vi "GeoData.vi"() -> ()   [LabVIEW 2017] (continued)
County\tH1\n40241\t21111\tLouisville\tKY\tJefferson County\tH1\n40207\t21111\tLouisville\tKY\tJefferson County\tH1\n40242\t21111\tLouisville\tKY\tJefferson County\tH1\n40272\t21111\tLouisville\tKY\tJefferson County\tH1\n40210\t21111\tLouisville\tKY\tJefferson County\tH1\n40270\t21111\tLouisville\tKY\tJefferson County\tH1\n40025\t21111\tGlenview\tKY\tJefferson County\tH1\n40027\t21111\tHarrods creek\tKY\tJefferson County\tH1\n40225\t21111\tLouisville\tKY\tJefferson County\tH1\n40281\t21111\tLouisville\tKY\tJefferson County\tH1\n40214\t21111\tLouisville\tKY\tJefferson County\tH1\n40257\t21111\tLouisville\tKY\tJefferson County\tH1\n40251\t21111\tLouisville\tKY\tJefferson County\tH1\n40292\t21111\tLouisville\tKY\tJefferson County\tH1\n40289\t21111\tLouisville\tKY\tJefferson County\tH1\n40177\t21111\tWest point\tKY\tJefferson County\tH1\n40216\t21111\tLouisville\tKY\tJefferson County\tH1\n40256\t21111\tLouisville\tKY\tJefferson County\tH1\n40291\t21111\tLouisville\tKY\tJefferson County\tH1\n40218\t21111\tLouisville\tKY\tJefferson County\tH1\n40217\t21111\tLouisville\tKY\tJefferson County\tH1\n40204\t21111\tLouisville\tKY\tJefferson County\tH1\n40056\t21111\tPewee valley\tKY\tJefferson County\tH1\n40250\t21111\tLouisville\tKY\tJefferson County\tH1\n40261\t21111\tLouisville\tKY\tJefferson County\tH1\n40018\t21111\tEastwood\tKY\tJefferson County\tH1\n40266\t21111\tLouisville\tKY\tJefferson County\tH1\n40285\t21111\tLouisville\tKY\tJefferson County\tH1\n40047\t21111\tMount washington\tKY\tJefferson County\tH1\n40059\t21111\tProspect\tKY\tJefferson County\tH1\n40219\t21111\tLouisville\tKY\tJefferson County\tH1\n40258\t21111\tLouisville\tKY\tJefferson County\tH1\n40205\t21111\tLouisville\tKY\tJefferson County\tH1\n40233\t21111\tLouisville\tKY\tJefferson County\tH1\n40255\t21111\tLouisville\tKY\tJefferson County\tH1\n40201\t21111\tLouisville\tKY\tJefferson County\tH1\n40202\t21111\tLouisville\tKY\tJefferson County\tH1\n40023\t21111\tFisherville\tKY\tJefferson County\tH1\n40245\t21111\tLouisville\tKY\tJefferson County\tH1\n40206\t21111\tLouisville\tKY\tJefferson County\tH1\n40228\t21111\tLouisville\tKY\tJefferson County\tH1\n40252\t21111\tLouisville\tKY\tJefferson County\tH1\n40268\t21111\tLouisville\tKY\tJefferson County\tH1\n40014\t21111\tCrestwood\tKY\tJefferson County\tH1\n40109\t21111\tBrooks\tKY\tJefferson County\tH1\n40118\t21111\tFairdale\tKY\tJefferson County\tH1\n40203\t21111\tLouisville\tKY\tJefferson County\tH1\n40211\t21111\tLouisville\tKY\tJefferson County\tH1\n40220\t21111\tLouisville\tKY\tJefferson County\tH1\n40243\t21111\tLouisville\tKY\tJefferson County\tH1\n40212\t21111\tLouisville\tKY\tJefferson County\tH1\n40215\t21111\tLouisville\tKY\tJefferson County\tH1\n40299\t21111\tLouisville\tKY\tJefferson County\tH1\n40253\t21111\tLouisville\tKY\tJefferson County\tH1\n40232\t21111\tLouisville\tKY\tJefferson County\tH1\n40283\t21111\tLouisville\tKY\tJefferson County\tH1\n40231\t21111\tLouisville\tKY\tJefferson County\tH1\n40223\t21111\tLouisville\tKY\tJefferson County\tH1\n40222\t21111\tLouisville\tKY\tJefferson County\tH1\n40208\t21111\tLouisville\tKY\tJefferson County\tH1\n40213\t21111\tLouisville\tKY\tJefferson County\tH1\n40221\t21111\tLouisville\tKY\tJefferson County\tH1\n40209\t21111\tLouisville\tKY\tJefferson County\tH1\n40383\t21113\tVersailles\tKY\tJessamine County\tH1\n40390\t21113\tWilmore\tKY\tJessamine County\tH1\n40340\t21113\tNicholasville\tKY\tJessamine County\tH1\n40515\t21113\tLexington\tKY\tJessamine County\tH1\n40339\t21113\tKeene\tKY\tJessamine County\tH1\n40356\t21113\tNicholasville\tKY\tJessamine County\tH1\n41255\t21115\tSitka\tKY\tJohnson County\tH1\n41240\t21115\tPaintsville\tKY\tJohnson County\tH1\n41238\t21115\tOil springs\tKY\tJohnson County\tH1\n41226\t21115\tKeaton\tKY\tJohnson County\tH1\n41256\t21115\tStaffordsville\tKY\tJohnson County\tH1\n41254\t21115\tRiver\tKY\tJohnson County\tH1\n41268\t21115\tWest van lear\tKY\tJohnson County\tH1\n41274\t21115\tWittensville\tKY\tJohnson County\tH1\n41465\t21115\tSalyersville\tKY\tJohnson County\tH1\n41219\t21115\tFlatgap\tKY\tJohnson County\tH1\n41159\t21115\tMartha\tKY\tJohnson County\tH1\n41260\t21115\tThelma\tKY\tJohnson County\tH1\n41204\t21115\tBoons camp\tKY\tJohnson County\tH1\n41265\t21115\tVan lear\tKY\tJohnson County\tH1\n41271\t21115\tWilliamsport\tKY\tJohnson County\tH1\n41257\t21115\tStambaugh\tKY\tJohnson County\tH1\n41263\t21115\tTutor key\tKY\tJohnson County\tH1\n41232\t21115\tLowmansville\tKY\tJohnson County\tH1\n41222\t21115\tHagerhill\tKY\tJohnson County\tH1\n41216\t21115\tEast point\tKY\tJohnson County\tH1\n41234\t21115\tMeally\tKY\tJohnson County\tH1\n41017\t21117\tFt mitchell\tKY\tKenton County\tH1\n41033\t21117\tDe mossville\tKY\tKenton County\tH1\n41015\t21117\tLatonia\tKY\tKenton County\tH1\n41018\t21117\tErlanger\tKY\tKenton County\tH1\n41030\t21117\tCrittenden\tKY\tKenton County\tH1\n41011\t21117\tCovington\tKY\tKenton County\tH1\n41063\t21117\tMorning view\tKY\tKenton County\tH1\n41053\t21117\tKenton\tKY\tKenton County\tH1\n41042\t21117\tFlorence\tKY\tKenton County\tH1\n41016\t21117\tCovington\tKY\tKenton County\tH1\n41094\t21117\tWalton\tKY\tKenton County\tH1\n41014\t21117\tCovington\tKY\tKenton County\tH1\n41012\t21117\tCovington\tKY\tKenton County\tH1\n41051\t21117\tIndependence\tKY\tKenton County\tH1\n45999\t21117\tCincinnati\tKY\tKenton County\tH1\n41339\t21119\tJackson\tKY\tKnott County\tH1\n41772\t21119\tVest\tKY\tKnott County\tH1\n41862\t21119\tTopmost\tKY\tKnott County\tH1\n41804\t21119\tBlackey\tKY\tKnott County\tH1\n41861\t21119\tRaven\tKY\tKnott County\tH1\n41859\t21119\tDema\tKY\tKnott County\tH1\n41722\t21119\tBulan\tKY\tKnott County\tH1\n41773\t21119\tVicco\tKY\tKnott County\tH1\n41828\t21119\tKite\tKY\tKnott County\tH1\n41725\t21119\tCarrie\tKY\tKnott County\tH1\n41743\t21119\tFisty\tKY\tKnott County\tH1\n41630\t21119\tGarrett\tKY\tKnott County\tH1\n41839\t21119\tMousie\tKY\tKnott County\tH1\n41834\t21119\tLittcarr\tKY\tKnott County\tH1\n41759\t21119\tSassafras\tKY\tKnott County\tH1\n41822\t21119\tHindman\tKY\tKnott County\tH1\n41701\t21119\tHazard\tKY\tKnott County\tH1\n41640\t21119\tHueysville\tKY\tKnott County\tH1\n41740\t21119\tEmmalena\tKY\tKnott County\tH1\n41847\t21119\tRedfox\tKY\tKnott County\tH1\n41836\t21119\tMallie\tKY\tKnott County\tH1\n41843\t21119\tPine top\tKY\tKnott County\tH1\n41817\t21119\tGarner\tKY\tKnott County\tH1\n41844\t21119\tPippa passes\tKY\tKnott County\tH1\n41831\t21119\tLeburn\tKY\tKnott County\tH1\n40903\t21121\tArtemus\tKY\tKnox County\tH1\n40982\t21121\tScalf\tKY\tKnox County\tH1\n40734\t21121\tGray\tKY\tKnox County\tH1\n40953\t21121\tHinkle\tKY\tKnox County\tH1\n40935\t21121\tFlat lick\tKY\tKnox County\tH1\n40997\t21121\tWalker\tKY\tKnox County\tH1\n40701\t21121\tCorbin\tKY\tKnox County\tH1\n40939\t21121\tFourmile\tKY\tKnox County\tH1\n40943\t21121\tGirdler\tKY\tKnox County\tH1\n40906\t21121\tBarbourville\tKY\tKnox County\tH1\n40923\t21121\tCannon\tKY\tKnox County\tH1\n40946\t21121\tGreen road\tKY\tKnox County\tH1\n40759\t21121\tRockholds\tKY\tKnox County\tH1\n40771\t21121\tWoodbine\tKY\tKnox County\tH1\n40915\t21121\tBimble\tKY\tKnox County\tH1\n40962\t21121\tManchester\tKY\tKnox County\tH1\n40763\t21121\tSiler\tKY\tKnox County\tH1\n40921\t21121\tBryants store\tKY\tKnox County\tH1\n40949\t21121\tHeidrick\tKY\tKnox County\tH1\n40995\t21121\tTrosper\tKY\tKnox County\tH1\n40051\t21123\tNew haven\tKY\tLarue County\tH1\n42716\t21123\tBuffalo\tKY\tLarue County\tH1\n42748\t21123\tHodgenville\tKY\tLarue County\tH1\n42757\t21123\tMagnolia\tKY\tLarue County\tH1\n40052\t21123\tNew hope\tKY\tLarue County\tH1\n42776\t21123\tSonora\tKY\tLarue County\tH1\n42764\t21123\tMount sherman\tKY\tLarue County\tH1\n42718\t21123\tCampbellsville\tKY\tLarue County\tH1\n42784\t21123\tUpton\tKY\tLarue County\tH1\n40740\t21125\tLily\tKY\tLaurel County\tH1\n40734\t21125\tGray\tKY\tLaurel County\tH1\n40701\t21125\tCorbin\tKY\tLaurel County\tH1\n40402\t21125\tAnnville\tKY\tLaurel County\tH1\n40729\t21125\tEast bernstadt\tKY\tLaurel County\tH1\n40906\t21125\tBarbourville\tKY\tLaurel County\tH1\n40755\t21125\tPittsburg\tKY\tLaurel County\tH1\n40744\t21125\tLondon\tKY\tLaurel County\tH1\n40741\t21125\tLondon\tKY\tLaurel County\tH1\n40962\t21125\tManchester\tKY\tLaurel County\tH1\n40750\t21125\tLondon\tKY\tLaurel County\tH1\n40456\t21125\tMount vernon\tKY\tLaurel County\tH1\n40737\t21125\tKeavy\tKY\tLaurel County\tH1\n40724\t21125\tBush\tKY\tLaurel County\tH1\n41124\t21127\tBlaine\tKY\tLawrence County\tH1\n41201\t21127\tAdams\tKY\tLawrence County\tH1\n41254\t21127\tRiver\tKY\tLawrence County\tH1\n41132\t21127\tDenton\tKY\tLawrence County\tH1\n41143\t21127\tGrayson\tKY\tLawrence County\tH1\n41159\t21127\tMartha\tKY\tLawrence County\tH1\n41180\t21127\tWebbville\tKY\tLawrence County\tH1\n41232\t21127\tLowmansville\tKY\tLawrence County\tH1\n41181\t21127\tWillard\tKY\tLawrence County\tH1\n41160\t21127\tMazie\tKY\tLawrence County\tH1\n41129\t21127\tCatlettsburg\tKY\tLawrence County\tH1\n41230\t21127\tLouisa\tKY\tLawrence County\tH1\n41264\t21127\tUlysses\tKY\tLawrence County\tH1\n41339\t21129\tJackson\tKY\tLee County\tH1\n41397\t21129\tZoe\tKY\tLee County\tH1\n41311\t21129\tBeattyville\tKY\tLee County\tH1\n41314\t21129\tBooneville\tKY\tLee County\tH1\n40336\t21129\tIrvine\tKY\tLee County\tH1\n41368\t21129\tSaint helens\tKY\tLee County\tH1\n41301\t21129\tCampton\tKY\tLee County\tH1\n41347\t21129\tLone\tKY\tLee County\tH1\n41365\t21129\tRogers\tKY\tLee County\tH1\n40858\t21131\tMozelle\tKY\tLeslie County\tH1\n41764\t21131\tSmilax\tKY\tLeslie County\tH1\n40914\t21131\tBig creek\tKY\tLeslie County\tH1\n41762\t21131\tSizerock\tKY\tLeslie County\tH1\n41723\t21131\tBusy\tKY\tLeslie County\tH1\n41777\t21131\tYeaddiss\tKY\tLeslie County\tH1\n40816\t21131\tChappell\tKY\tLeslie County\tH1\n41766\t21131\tThousandsticks\tKY\tLeslie County\tH1\n40818\t21131\tCoalgood\tKY\tLeslie County\tH1\n40803\t21131\tAsher\tKY\tLeslie County\tH1\n41776\t21131\tWooton\tKY\tLeslie County\tH1\n40972\t21131\tOneida\tKY\tLeslie County\tH1\n40868\t21131\tStinnett\tKY\tLeslie County\tH1\n41775\t21131\tWendover\tKY\tLeslie County\tH1\n40840\t21131\tHelton\tKY\tLeslie County\tH1\n40827\t21131\tEssie\tKY\tLeslie County\tH1\n40844\t21131\tHoskinston\tKY\tLeslie County\tH1\n40874\t21131\tWarbranch\tKY\tLeslie County\tH1\n40810\t21131\tBledsoe\tKY\tLeslie County\tH1\n41714\t21131\tBear branch\tKY\tLeslie County\tH1\n41754\t21131\tKrypton\tKY\tLeslie County\tH1\n40808\t21131\tBig laurel\tKY\tLeslie County\tH1\n40979\t21131\tRoark\tKY\tLeslie County\tH1\n41749\t21131\tHyden\tKY\tLeslie County\tH1\n41833\t21133\tLinefork\tKY\tLetcher County\tH1\n41858\t21133\tWhitesburg\tKY\tLetcher County\tH1\n40826\t21133\tEolia\tKY\tLetcher County\tH1\n41835\t21133\tMc roberts\tKY\tLetcher County\tH1\n41804\t21133\tBlackey\tKY\tLetcher County\tH1\n41832\t21133\tLetcher\tKY\tLetcher County\tH1\n40823\t21133\tCumberland\tKY\tLetcher County\tH1\n41845\t21133\tPremium\tKY\tLetcher County\tH1\n41819\t21133\tGordon\tKY\tLetcher County\tH1\n41840\t21133\tNeon\tKY\tLetcher County\tH1\n41812\t21133\tDeane\tKY\tLetcher County\tH1\n41821\t21133\tHallie\tKY\tLetcher County\tH1\n41838\t21133\tMillstone\tKY\tLetcher County\tH1\n41837\t21133\tMayking\tKY\tLetcher County\tH1\n41855\t21133\tThornton\tKY\tLetcher County\tH1\n41815\t21133\tErmine\tKY\tLetcher County\tH1\n41849\t21133\tSeco\tKY\tLetcher County\tH1\n41537\t21133\tJenkins\tKY\tLetcher County\tH1\n41824\t21133\tIsom\tKY\tLetcher County\tH1\n41848\t21133\tRoxana\tKY\tLetcher County\tH1\n41826\t21133\tJeremiah\tKY\tLetcher County\tH1\n41825\t21133\tJackhorn\tKY\tLetcher County\tH1\n40862\t21133\tPartridge\tKY\tLetcher County\tH1\n41517\t21133\tBurdine\tKY\tLetcher County\tH1\n41731\t21133\tCornettsville\tKY\tLetcher County\tH1\n41810\t21133\tCromona\tKY\tLetcher County\tH1\n41056\t21135\tMaysville\tKY\tLewis County\tH1\n41093\t21135\tWallingford\tKY\tLewis County\tH1\n41135\t21135\tEmerson\tKY\tLewis County\tH1\n41189\t21135\tTollesboro\tKY\tLewis County\tH1\n41174\t21135\tSouth portsmouth\tKY\tLewis County\tH1\n41179\t21135\tVanceburg\tKY\tLewis County\tH1\n41175\t21135\tSouth shore\tKY\tLewis County\tH1\n41141\t21135\tGarrison\tKY\tLewis County\tH1\n41164\t21135\tOlive hill\tKY\tLewis County\tH1\n41166\t21135\tQuincy\tKY\tLewis County\tH1\n40437\t21137\tHustonville\tKY\tLincoln County\tH1\n40409\t21137\tBrodhead\tKY\tLincoln County\tH1\n40442\t21137\tKings mountain\tKY\tLincoln County\tH1\n40484\t21137\tStanford\tKY\tLincoln County\tH1\n40444\t21137\tLancaster\tKY\tLincoln County\tH1\n40489\t21137\tWaynesburg\tKY\tLincoln County\tH1\n40440\t21137\tJunction city\tKY\tLincoln County\tH1\n40422\t21137\tDanville\tKY\tLincoln County\tH1\n42567\t21137\tEubank\tKY\tLincoln County\tH1\n40448\t21137\tMc kinney\tKY\tLincoln County\tH1\n40419\t21137\tCrab orchard\tKY\tLincoln County\tH1\n40461\t21137\tPaint lick\tKY\tLincoln County\tH1\n42081\t21139\tSmithland\tKY\tLivingston County\tH1\n42028\t21139\tBurna\tKY\tLivingston County\tH1\n42078\t21139\tSalem\tKY\tLivingston County\tH1\n42064\t21139\tMarion\tKY\tLivingston County\tH1\n42045\t21139\tGrand rivers\tKY\tLivingston County\tH1\n42047\t21139\tHampton\tKY\tLivingston County\tH1\n42058\t21139\tLedbetter\tKY\tLivingston County\tH1\n42083\t21139\tTiline\tKY\tLivingston County\tH1\n42265\t21141\tOlmstead\tKY\tLogan County\tH1\n42339\t21141\tDunmor\tKY\tLogan County\tH1\n42206\t21141\tAuburn\tKY\tLogan County\tH1\n42276\t21141\tRussellville\tKY\tLogan County\tH1\n42256\t21141\tLewisburg\tKY\tLogan County\tH1\n42202\t21141\tAdairville\tKY\tLogan County\tH1\n42274\t21141\tRockfield\tKY\tLogan County\tH1\n42170\t21141\tWoodburn\tKY\tLogan County\tH1\n42204\t21141\tAllensville\tKY\tLogan County\tH1\n42261\t21141\tMorgantown\tKY\tLogan County\tH1\n42038\t21143\tEddyville\tKY\tLyon County\tH1\n42211\t21143\tCadiz\tKY\tLyon County\tH1\n42411\t21143\tFredonia\tKY\tLyon County\tH1\n42445\t21143\tPrinceton\tKY\tLyon County\tH1\n42045\t21143\tGrand rivers\tKY\tLyon County\tH1\n42055\t21143\tKuttawa\tKY\tLyon County\tH1\n42001\t21145\tPaducah\tKY\tMcCracken County\tH1\n42003\t21145\tPaducah\tKY\tMcCracken County\tH1\n42053\t21145\tKevil\tKY\tMcCracken County\tH1\n42086\t21145\tWest paducah\tKY\tMcCracken County\tH1\n42029\t21145\tCalvert city\tKY\tMcCracken County\tH1\n42002\t21145\tPaducah\tKY\tMcCracken County\tH1\n42027\t21145\tBoaz\tKY\tMcCracken County\tH1\n42082\t21145\tSymsonia\tKY\tMcCracken County\tH1\n42069\t21145\tMelber\tKY\tMcCracken County\tH1\n40769\t21147\tWilliamsburg\tKY\tMcCreary County\tH1\n42631\t21147\tMarshes siding\tKY\tMcCreary County\tH1\n42634\t21147\tParkers lake\tKY\tMcCreary County\tH1\n42635\t21147\tPine knot\tKY\tMcCreary County\tH1\n42647\t21147\tStearns\tKY\tMcCreary County\tH1\n42649\t21147\tStrunk\tKY\tMcCreary County\tH1\n42653\t21147\tWhitley city\tKY\tMcCreary County\tH1\n42638\t21147\tRevelo\tKY\tMcCreary County\tH1\n42352\t21149\tLivermore\tKY\tMcLean County\tH1\n42330\t21149\tCentral city\tKY\tMcLean County\tH1\n42350\t21149\tIsland\tKY\tMcLean County\tH1\n42327\t21149\tCalhoun\tKY\tMcLean County\tH1\n42372\t21149\tSacramento\tKY\tMcLean County\tH1\n42371\t21149\tRumsey\tKY\tMcLean County\tH1\n42301\t21149\tOwensboro\tKY\tMcLean County\tH1\n42322\t21149\tBeech grove\tKY\tMcLean County\tH1\n42376\t21149\tUtica\tKY\tMcLean County\tH1\n40403\t21151\tBerea\tKY\tMadison County\tH1\n40475\t21151\tRichmond\tKY\tMadison County\tH1\n40405\t21151\tBighill\tKY\tMadison County\tH1\n40447\t21151\tMc kee\tKY\tMadison County\tH1\n40456\t21151\tMount vernon\tKY\tMadison County\tH1\n40385\t21151\tWaco\tKY\tMadison County\tH1\n40476\t21151\tRichmond\tKY\tMadison County\tH1\n40461\t21151\tPaint lick\tKY\tMadison County\tH1\n41464\t21153\tRoyalton\tKY\tMagoffin County\tH1\n41465\t21153\tSalyersville\tKY\tMagoffin County\tH1\n41472\t21153\tWest liberty\tKY\tMagoffin County\tH1\n41332\t21153\tHazel green\tKY\tMagoffin County\tH1\n41632\t21153\tGunlock\tKY\tMagoffin County\tH1\n41426\t21153\tFalcon\tKY\tMagoffin County\tH1\n40037\t21155\tLoretto\tKY\tMarion County\tH1\n40069\t21155\tSpringfield\tKY\tMarion County\tH1\n40009\t21155\tBradfordsville\tKY\tMarion County\tH1\n40052\t21155\tNew hope\tKY\tMarion County\tH1\n42743\t21155\tGreensburg\tKY\tMarion County\tH1\n40049\t21155\tNerinx\tKY\tMarion County\tH1\n40033\t21155\tLebanon\tKY\tMarion County\tH1\n40062\t21155\tSaint francis\tKY\tMarion County\tH1\n40063\t21155\tSaint mary\tKY\tMarion County\tH1\n40060\t21155\tRaywick\tKY\tMarion County\tH1\n42718\t21155\tCampbellsville\tKY\tMarion County\tH1\n40328\t21155\tGravel switch\tKY\tMarion County\tH1\n42048\t21157\tHardin\tKY\tMarshall County\tH1\n42054\t21157\tKirksey\tKY\tMarshall County\tH1\n42003\t21157\tPaducah\tKY\tMarshall County\tH1\n42044\t21157\tGilbertsville\tKY\tMarshall County\tH1\n42025\t21157\tBenton\tKY\tMarshall County\tH1\n42029\t21157\tCalvert city\tKY\tMarshall County\tH1\n42082\t21157\tSymsonia\tKY\tMarshall County\tH1\n42066\t21157\tMayfield\tKY\tMarshall County\tH1\n42036\t21157\tDexter\tKY\tMarshall County\tH1\n41267\t21159\tWarfield\tKY\tMartin County\tH1\n41514\t21159\tBelfry\tKY\tMartin County\tH1\n41231\t21159\tLovely\tKY\tMartin County\tH1\n41203\t21159\tBeauty\tKY\tMartin County\tH1\n41214\t21159\tDebord\tKY\tMartin County\tH1\n41262\t21159\tTomahawk\tKY\tMartin County\tH1\n41250\t21159\tPilgrim\tKY\tMartin County\tH1\n41230\t21159\tLouisa\tKY\tMartin County\tH1\n41224\t21159\tInez\tKY\tMartin County\tH1\n41044\t21161\tGermantown\tKY\tMason County\tH1\n41056\t21161\tMaysville\tKY\tMason County\tH1\n41002\t21161\tAugusta\tKY\tMason County\tH1\n41034\t21161\tDover\tKY\tMason County\tH1\n41062\t21161\tMinerva\tKY\tMason County\tH1\n41055\t21161\tMayslick\tKY\tMason County\tH1\n41039\t21161\tEwing\tKY\tMason County\tH1\n41041\t21161\tFlemingsburg\tKY\tMason County\tH1\n41096\t21161\tWashington\tKY\tMason County\tH1\n40146\t21163\tIrvington\tKY\tMeade County\tH1\n40161\t21163\tRhodelia\tKY\tMeade County\tH1\n40157\t21163\tPayneville\tKY\tMeade County\tH1\n40108\t21163\tBrandenburg\tKY\tMeade County\tH1\n40121\t21163\tFort knox\tKY\tMeade County\tH1\n40117\t21163\tEkron\tKY\tMeade County\tH1\n40155\t21163\tMuldraugh\tKY\tMeade County\tH1\n40175\t21163\tVine grove\tKY\tMeade County\tH1\n40171\t21163\tUnion star\tKY\tMeade County\tH1\n40142\t21163\tGuston\tKY\tMeade County\tH1\n40176\t21163\tWebster\tKY\tMeade County\tH1\n40104\t21163\tBattletown\tKY\tMeade County\tH1\n40346\t21165\tMeans\tKY\tMenifee County\tH1\n40316\t21165\tDenniston\tKY\tMenifee County\tH1\n40387\t21165\tWellington\tKY\tMenifee County\tH1\n40380\t21165\tStanton\tKY\tMenifee County\tH1\n41472\t21165\tWest liberty\tKY\tMenifee County\tH1\n40371\t21165\tSalt lick\tKY\tMenifee County\tH1\n40322\t21165\tFrenchburg\tKY\tMenifee County\tH1\n40468\t21167\tPerryville\tKY\tMercer County\tH1\n40444\t21167\tLancaster\tKY\tMercer County\tH1\n40078\t21167\tWillisburg\tKY\tMercer County\tH1\n40342\t21167\tLawrenceburg\tKY\tMercer County\tH1\n40310\t21167\tBurgin\tKY\tMercer County\tH1\n40330\t21167\tHarrodsburg\tKY\tMercer County\tH1\n40372\t21167\tSalvisa\tKY\tMercer County\tH1\n42166\t21169\tSummer shade\tKY\tMetcalfe County\tH1\n42129\t21169\tEdmonton\tKY\tMetcalfe County\tH1\n42749\t21169\tHorse cave\tKY\tMetcalfe County\tH1\n42715\t21169\tBreeding\tKY\tMetcalfe County\tH1\n42717\t21169\tBurkesville\tKY\tMetcalfe County\tH1\n42154\t21169\tKnob lick\tKY\tMetcalfe County\tH1\n42141\t21169\tGlasgow\tKY\tMetcalfe County\tH1\n42124\t21169\tBeaumont\tKY\tMetcalfe County\tH1\n42214\t21169\tCenter\tKY\tMetcalfe County\tH1\n42746\t21169\tHardyville\tKY\tMetcalfe County\tH1\n42140\t21171\tGamaliel\tKY\tMonroe County\tH1\n42133\t21171\tFountain run\tKY\tMonroe County\tH1\n42166\t21171\tSummer shade\tKY\tMonroe County\tH1\n42151\t21171\tHestand\tKY\tMonroe County\tH1\n42164\t21171\tScottsville\tKY\tMonroe County\tH1\n42157\t21171\tMount hermon\tKY\tMonroe County\tH1\n42167\t21171\tTompkinsville\tKY\tMonroe County\tH1\n40353\t21173\tMount sterling\tKY\tMontgomery County\tH1\n40346\t21173\tMeans\tKY\tMontgomery County\tH1\n40391\t21173\tWinchester\tKY\tMontgomery County\tH1\n40334\t21173\tHope\tKY\tMontgomery County\tH1\n40361\t21173\tParis\tKY\tMontgomery County\tH1\n40337\t21173\tJeffersonville\tKY\tMontgomery County\tH1\n40360\t21173\tOwingsville\tKY\tMontgomery County\tH1\n41421\t21175\tElkfork\tKY\tMorgan County\tH1\n41451\t21175\tMalone\tKY\tMorgan County\tH1\n41465\t21175\tSalyersville\tKY\tMorgan County\tH1\n41219\t21175\tFlatgap\tKY\tMorgan County\tH1\n40387\t21175\tWellington\tKY\tMorgan County\tH1\n41171\t21175\tSandy hook\tKY\tMorgan County\tH1\n41425\t21175\tEzel\tKY\tMorgan County\tH1\n41149\t21175\tIsonville\tKY\tMorgan County\tH1\n41472\t21175\tWest liberty\tKY\tMorgan County\tH1\n41332\t21175\tHazel green\tKY\tMorgan County\tH1\n41413\t21175\tCrockett\tKY\tMorgan County\tH1\n41408\t21175\tCannel city\tKY\tMorgan County\tH1\n41352\t21175\tMize\tKY\tMorgan County\tH1\n42367\t21177\tPowderly\tKY\tMuhlenberg County\tH1\n42374\t21177\tSouth carrollton\tKY\tMuhlenberg County\tH1\n42339\t21177\tDunmor\tKY\tMuhlenberg County\tH1\n42345\t21177\tGreenville\tKY\tMuhlenberg County\tH1\n42325\t21177\tBremen\tKY\tMuhlenberg County\tH1\n42321\t21177\tBeech creek\tKY\tMuhlenberg County\tH1\n42324\t21177\tBelton\tKY\tMuhlenberg County\tH1\n42344\t21177\tGraham\tKY\tMuhlenberg County\tH1\n42256\t21177\tLewisburg\tKY\tMuhlenberg County\tH1\n42330\t21177\tCentral city\tKY\tMuhlenberg County\tH1\n42337\t21177\tDrakesboro\tKY\tMuhlenberg County\tH1\n42372\t21177\tSacramento\tKY\tMuhlenberg County\tH1\n42326\t21177\tBrowder\tKY\tMuhlenberg County\tH1\n42220\t21177\tElkton\tKY\tMuhlenberg County\tH1\n42323\t21177\tBeechmont\tKY\tMuhlenberg County\tH1\n42332\t21177\tCleaton\tKY\tMuhlenberg County\tH1\n42464\t21177\tWhite plains\tKY\tMuhlenberg County\tH1\n40051\t21179\tNew haven\tKY\tNelson County\tH1\n40037\t21179\tLoretto\tKY\tNelson County\tH1\n40069\t21179\tSpringfield\tKY\tNelson County\tH1\n40012\t21179\tChaplin\tKY\tNelson County\tH1\n42748\t21179\tHodgenville\tKY\tNelson County\tH1\n40052\t21179\tNew hope\tKY\tNelson County\tH1\n40020\t21179\tFairfield\tKY\tNelson County\tH1\n40008\t21179\tBloomfield\tKY\tNelson County\tH1\n40071\t21179\tTaylorsville\tKY\tNelson County\tH1\n40004\t21179\tBardstown\tKY\tNelson County\tH1\n40013\t21179\tCoxs creek\tKY\tNelson County\tH1\n40107\t21179\tBoston\tKY\tNelson County\tH1\n40048\t21179\tNazareth\tKY\tNelson County\tH1\n40311\t21181\tCarlisle\tKY\tNicholas County\tH1\n41031\t21181\tCynthiana\tKY\tNicholas County\tH1\n40350\t21181\tMoorefield\tKY\tNicholas County\tH1\n40361\t21181\tParis\tKY\tNicholas County\tH1\n41039\t21181\tEwing\tKY\tNicholas County\tH1\n40374\t21181\tSharpsburg\tKY\tNicholas County\tH1\n42354\t21183\tMc henry\tKY\tOhio County\tH1\n42352\t21183\tLivermore\tKY\tOhio County\tH1\n42361\t21183\tOlaton\tKY\tOhio County\tH1\n42328\t21183\tCentertown\tKY\tOhio County\tH1\n42369\t21183\tRockport\tKY\tOhio County\tH1\n42349\t21183\tHorse branch\tKY\tOhio County\tH1\n42343\t21183\tFordsville\tKY\tOhio County\tH1\n42333\t21183\tCromwell\tKY\tOhio County\tH1\n42338\t21183\tDundee\tKY\tOhio County\tH1\n42370\t21183\tRosine\tKY\tOhio County\tH1\n42366\t21183\tPhilpot\tKY\tOhio County\tH1\n42368\t21183\tReynolds station\tKY\tOhio County\tH1\n42378\t21183\tWhitesville\tKY\tOhio County\tH1\n42320\t21183\tBeaver dam\tKY\tOhio County\tH1\n42347\t21183\tHartford\tKY\tOhio County\tH1\n40119\t21183\tFalls of rough\tKY\tOhio County\tH1\n42376\t21183\tUtica\tKY\tOhio County\tH1\n40241\t21185\tLouisville\tKY\tOldham County\tH1\n40010\t21185\tBuckner\tKY\tOldham County\tH1\n40032\t21185\tLa grange\tKY\tOldham County\tH1\n40077\t21185\tWestport\tKY\tOldham County\tH1\n40056\t21185\tPewee valley\tKY\tOldham County\tH1\n40059\t21185\tProspect\tKY\tOldham County\tH1\n40026\t21185\tGoshen\tKY\tOldham County\tH1\n40245\t21185\tLouisville\tKY\tOldham County\tH1\n40014\t21185\tCrestwood\tKY\tOldham County\tH1\n40068\t21185\tSmithfield\tKY\tOldham County\tH1\n40031\t21185\tLa grange\tKY\tOldham County\tH1\n40065\t21185\tShelbyville\tKY\tOldham County\tH1\n40055\t21185\tPendleton\tKY\tOldham County\tH1\n41046\t21187\tGlencoe\tKY\tOwen County\tH1\n40355\t21187\tNew liberty\tKY\tOwen County\tH1\n41098\t21187\tWorthville\tKY\tOwen County\tH1\n41052\t21187\tJonesville\tKY\tOwen County\tH1\n41083\t21187\tSanders\tKY\tOwen County\tH1\n40379\t21187\tStamping ground\tKY\tOwen County\tH1\n41086\t21187\tSparta\tKY\tOwen County\tH1\n41035\t21187\tDry ridge\tKY\tOwen County\tH1\n40359\t21187\tOwenton\tKY\tOwen County\tH1\n40363\t21187\tPerry park\tKY\tOwen County\tH1\n41010\t21187\tCorinth\tKY\tOwen County\tH1\n41311\t21189\tBeattyville\tKY\tOwsley County\tH1\n41351\t21189\tMistletoe\tKY\tOwsley County\tH1\n41314\t21189\tBooneville\tKY\tOwsley County\tH1\n40486\t21189\tTyner\tKY\tOwsley County\tH1\n40447\t21189\tMc kee\tKY\tOwsley County\tH1\n41364\t21189\tRicetown\tKY\tOwsley County\tH1\n41386\t21189\tVincent\tKY\tOwsley County\tH1\n41097\t21191\tWilliamstown\tKY\tPendleton County\tH1\n41043\t21191\tFoster\tKY\tPendleton County\tH1\n41033\t21191\tDe mossville\tKY\tPendleton County\tH1\n41003\t21191\tBerry\tKY\tPendleton County\tH1\n41030\t21191\tCrittenden\tKY\tPendleton County\tH1\n41035\t21191\tDry ridge\tKY\tPendleton County\tH1\n41007\t21191\tCalifornia\tKY\tPendleton County\tH1\n41040\t21191\tFalmouth\tKY\tPendleton County\tH1\n41006\t21191\tButler\tKY\tPendleton County\tH1\n41339\t21193\tJackson\tKY\tPerry County\tH1\n41721\t21193\tBuckhorn\tKY\tPerry County\tH1\n41763\t21193\tSlemp\tKY\tPerry County\tH1\n41735\t21193\tDelphia\tKY\tPerry County\tH1\n41746\t21193\tHappy\tKY\tPerry County\tH1\n41774\t21193\tViper\tKY\tPerry County\tH1\n41745\t21193\tGays creek\tKY\tPerry County\tH1\n41760\t21193\tScuddy\tKY\tPerry County\tH1\n41713\t21193\tAvawam\tKY\tPerry County\tH1\n41723\t21193\tBusy\tKY\tPerry County\tH1\n41778\t21193\tYerkes\tKY\tPerry County\tH1\n41729\t21193\tCombs\tKY\tPerry County\tH1\n41719\t21193\tBonnyman\tKY\tPerry County\tH1\n41712\t21193\tAry\tKY\tPerry County\tH1\n41722\t21193\tBulan\tKY\tPerry County\tH1\n41773\t21193\tVicco\tKY\tPerry County\tH1\n40972\t21193\tOneida\tKY\tPerry County\tH1\n41751\t21193\tJeff\tKY\tPerry County\tH1\n41727\t21193\tChavies\tKY\tPerry County\tH1\n41739\t21193\tDwarf\tKY\tPerry County\tH1\n41736\t21193\tDice\tKY\tPerry County\tH1\n41348\t21193\tLost creek\tKY\tPerry County\tH1\n41701\t21193\tHazard\tKY\tPerry County\tH1\n41754\t21193\tKrypton\tKY\tPerry County\tH1\n41731\t21193\tCornettsville\tKY\tPerry County\tH1\n41367\t21193\tRowdy\tKY\tPerry County\tH1\n41519\t21195\tCanada\tKY\tPike County\tH1\n41544\t21195\tMc carr\tKY\tPike County\tH1\n41501\t21195\tPikeville\tKY\tPike County\tH1\n41514\t21195\tBelfry\tKY\tPike County\tH1\n41562\t21195\tShelbiana\tKY\tPike County\tH1\n41527\t21195\tForest hills\tKY\tPike County\tH1\n41557\t21195\tRaccoon\tKY\tPike County\tH1\n41560\t21195\tRobinson creek\tKY\tPike County\tH1\n41561\t21195\tRockhouse\tKY\tPike County\tH1\n41534\t21195\tHellier\tKY\tPike County\tH1\n41566\t21195\tSteele\tKY\tPike County\tH1\n41513\t21195\tBelcher\tKY\tPike County\tH1\n41524\t21195\tFedscreek\tKY\tPike County\tH1\n41572\t21195\tVirgie\tKY\tPike County\tH1\n41512\t21195\tAshcamp\tKY\tPike County\tH1\n41503\t21195\tSouth williamson\tKY\tPike County\tH1\n41558\t21195\tRansom\tKY\tPike County\tH1\n41555\t21195\tPinsonfork\tKY\tPike County\tH1\n41549\t21195\tMyra\tKY\tPike County\tH1\n41520\t21195\tDorton\tKY\tPike County\tH1\n41563\t21195\tShelby gap\tKY\tPike County\tH1\n41539\t21195\tKimper\tKY\tPike County\tH1\n41548\t21195\tMouthcard\tKY\tPike County\tH1\n41653\t21195\tPrestonsburg\tKY\tPike County\tH1\n41502\t21195\tPikeville\tKY\tPike County\tH1\n41528\t21195\tFreeburn\tKY\tPike County\tH1\n41568\t21195\tStopover\tKY\tPike County\tH1\n41537\t21195\tJenkins\tKY\tPike County\tH1\n41547\t21195\tMajestic\tKY\tPike County\tH1\n41543\t21195\tMc andrews\tKY\tPike County\tH1\n41526\t21195\tFords branch\tKY\tPike County\tH1\n41522\t21195\tElkhorn city\tKY\tPike County\tH1\n41531\t21195\tHardy\tKY\tPike County\tH1\n41553\t21195\tPhelps\tKY\tPike County\tH1\n41554\t21195\tPhyllis\tKY\tPike County\tH1\n41659\t21195\tStanville\tKY\tPike County\tH1\n41535\t21195\tHuddy\tKY\tPike County\tH1\n41559\t21195\tRegina\tKY\tPike County\tH1\n41571\t21195\tVarney\tKY\tPike County\tH1\n41567\t21195\tStone\tKY\tPike County\tH1\n41605\t21195\tBetsy layne\tKY\tPike County\tH1\n41564\t21195\tSidney\tKY\tPike County\tH1\n41538\t21195\tJonancy\tKY\tPike County\tH1\n41540\t21195\tLick creek\tKY\tPike County\tH1\n41542\t21195\tLookout\tKY\tPike County\tH1\n40376\t21197\tSlade\tKY\tPowell County\tH1\n40312\t21197\tClay city\tKY\tPowell County\tH1\n40387\t21197\tWellington\tKY\tPowell County\tH1\n41360\t21197\tPine ridge\tKY\tPowell County\tH1\n40380\t21197\tStanton\tKY\tPowell County\tH1\n41301\t21197\tCampton\tKY\tPowell County\tH1\n40337\t21197\tJeffersonville\tKY\tPowell County\tH1\n40472\t21197\tRavenna\tKY\tPowell County\tH1\n40409\t21199\tBrodhead\tKY\tPulaski County\tH1\n42533\t21199\tFerguson\tKY\tPulaski County\tH1\n40489\t21199\tWaynesburg\tKY\tPulaski County\tH1\n42642\t21199\tRussell springs\tKY\tPulaski County\tH1\n42558\t21199\tTateville\tKY\tPulaski County\tH1\n42503\t21199\tSomerset\tKY\tPulaski County\tH1\n42633\t21199\tMonticello\tKY\tPulaski County\tH1\n42544\t21199\tNancy\tKY\tPulaski County\tH1\n42564\t21199\tWest somerset\tKY\tPulaski County\tH1\n42567\t21199\tEubank\tKY\tPulaski County\tH1\n42519\t21199\tBurnside\tKY\tPulaski County\tH1\n40456\t21199\tMount vernon\tKY\tPulaski County\tH1\n42553\t21199\tScience hill\tKY\tPulaski County\tH1\n42502\t21199\tSomerset\tKY\tPulaski County\tH1\n40419\t21199\tCrab orchard\tKY\tPulaski County\tH1\n42501\t21199\tSomerset\tKY\tPulaski County\tH1\n42518\t21199\tBronston\tKY\tPulaski County\tH1\n41031\t21201\tCynthiana\tKY\tRobertson County\tH1\n41044\t21201\tGermantown\tKY\tRobertson County\tH1\n41004\t21201\tBrooksville\tKY\tRobertson County\tH1\n41055\t21201\tMayslick\tKY\tRobertson County\tH1\n41064\t21201\tMount olivet\tKY\tRobertson County\tH1\n40403\t21203\tBerea\tKY\tRockcastle County\tH1\n40409\t21203\tBrodhead\tKY\tRockcastle County\tH1\n40492\t21203\tWildie\tKY\tRockcastle County\tH1\n40473\t21203\tRenfro valley\tKY\tRockcastle County\tH1\n40460\t21203\tOrlando\tKY\tRockcastle County\tH1\n40447\t21203\tMc kee\tKY\tRockcastle County\tH1\n40456\t21203\tMount vernon\tKY\tRockcastle County\tH1\n40419\t21203\tCrab orchard\tKY\tRockcastle County\tH1\n40445\t21203\tLivingston\tKY\tRockcastle County\tH1\n40317\t21205\tElliottville\tKY\tRowan County\tH1\n41049\t21205\tHillsboro\tKY\tRowan County\tH1\n41171\t21205\tSandy hook\tKY\tRowan County\tH1\n40313\t21205\tClearfield\tKY\tRowan County\tH1\n40351\t21205\tMorehead\tKY\tRowan County\tH1\n41472\t21205\tWest liberty\tKY\tRowan County\tH1\n40371\t21205\tSalt lick\tKY\tRowan County\tH1\n40319\t21205\tFarmers\tKY\tRowan County\tH1\n41164\t21205\tOlive hill\tKY\tRowan County\tH1\n42642\t21207\tRussell springs\tKY\tRussell County\tH1\n42741\t21207\tGlens fork\tKY\tRussell County\tH1\n42602\t21207\tAlbany\tKY\tRussell County\tH1\n42539\t21207\tLiberty\tKY\tRussell County\tH1\n42633\t21207\tMonticello\tKY\tRussell County\tH1\n42544\t21207\tNancy\tKY\tRussell County\tH1\n42629\t21207\tJamestown\tKY\tRussell County\tH1\n42528\t21207\tDunnville\tKY\tRussell County\tH1\n40370\t21209\tSadieville\tKY\tScott County\tH1\n40324\t21209\tGeorgetown\tKY\tScott County\tH1\n40347\t21209\tMidway\tKY\tScott County\tH1\n40379\t21209\tStamping ground\tKY\tScott County\tH1\n40511\t21209\tLexington\tKY\tScott County\tH1\n40361\t21209\tParis\tKY\tScott County\tH1\n41010\t21209\tCorinth\tKY\tScott County\tH1\n40019\t21211\tEminence\tKY\tShelby County\tH1\n40046\t21211\tMount eden\tKY\tShelby County\tH1\n40067\t21211\tSimpsonville\tKY\tShelby County\tH1\n40056\t21211\tPewee valley\tKY\tShelby County\tH1\n40601\t21211\tFrankfort\tKY\tShelby County\tH1\n40342\t21211\tLawrenceburg\tKY\tShelby County\tH1\n40066\t21211\tShelbyville\tKY\tShelby County\tH1\n40071\t21211\tTaylorsville\tKY\tShelby County\tH1\n40076\t21211\tWaddy\tKY\tShelby County\tH1\n40023\t21211\tFisherville\tKY\tShelby County\tH1\n40245\t21211\tLouisville\tKY\tShelby County\tH1\n40014\t21211\tCrestwood\tKY\tShelby County\tH1\n40057\t21211\tPleasureville\tKY\tShelby County\tH1\n40068\t21211\tSmithfield\tKY\tShelby County\tH1\n40022\t21211\tFinchville\tKY\tShelby County\tH1\n40065\t21211\tShelbyville\tKY\tShelby County\tH1\n40003\t21211\tBagdad\tKY\tShelby County\tH1\n42104\t21213\tBowling green\tKY\tSimpson County\tH1\n42206\t21213\tAuburn\tKY\tSimpson County\tH1\n42134\t21213\tFranklin\tKY\tSimpson County\tH1\n42276\t21213\tRussellville\tKY\tSimpson County\tH1\n42202\t21213\tAdairville\tKY\tSimpson County\tH1\n42170\t21213\tWoodburn\tKY\tSimpson County\tH1\n40046\t21215\tMount eden\tKY\tSpencer County\tH1\n40047\t21215\tMount washington\tKY\tSpencer County\tH1\n40008\t21215\tBloomfield\tKY\tSpencer County\tH1\n40342\t21215\tLawrenceburg\tKY\tSpencer County\tH1\n40071\t21215\tTaylorsville\tKY\tSpencer County\tH1\n40076\t21215\tWaddy\tKY\tSpencer County\tH1\n40023\t21215\tFisherville\tKY\tSpencer County\tH1\n40013\t21215\tCoxs creek\tKY\tSpencer County\tH1\n42716\t21217\tBuffalo\tKY\tTaylor County\tH1\n40009\t21217\tBradfordsville\tKY\tTaylor County\tH1\n42728\t21217\tColumbia\tKY\tTaylor County\tH1\n42743\t21217\tGreensburg\tKY\tTaylor County\tH1\n40033\t21217\tLebanon\tKY\tTaylor County\tH1\n42758\t21217\tMannsville\tKY\tTaylor County\tH1\n42733\t21217\tElk horn\tKY\tTaylor County\tH1\n42718\t21217\tCampbellsville\tKY\tTaylor County\tH1\n42265\t21219\tOlmstead\tKY\tTodd County\tH1\n42345\t21219\tGreenville\tKY\tTodd County\tH1\n42266\t21219\tPembroke\tKY\tTodd County\tH1\n42280\t21219\tSharon grove\tKY\tTodd County\tH1\n42276\t21219\tRussellville\tKY\tTodd County\tH1\n42256\t21219\tLewisburg\tKY\tTodd County\tH1\n42221\t21219\tFairview\tKY\tTodd County\tH1\n42234\t21219\tGuthrie\tKY\tTodd County\tH1\n42220\t21219\tElkton\tKY\tTodd County\tH1\n42216\t21219\tClifty\tKY\tTodd County\tH1\n42204\t21219\tAllensville\tKY\tTodd County\tH1\n42240\t21219\tHopkinsville\tKY\tTodd County\tH1\n42286\t21219\tTrenton\tKY\tTodd County\tH1\n42038\t21221\tEddyville\tKY\tTrigg County\tH1\n42211\t21221\tCadiz\tKY\tTrigg County\tH1\n42215\t21221\tCerulean\tKY\tTrigg County\tH1\n42445\t21221\tPrinceton\tKY\tTrigg County\tH1\n42236\t21221\tHerndon\tKY\tTrigg County\tH1\n42232\t21221\tGracey\tKY\tTrigg County\tH1\n40006\t21223\tBedford\tKY\tTrimble County\tH1\n40045\t21223\tMilton\tKY\tTrimble County\tH1\n40011\t21223\tCampbellsburg\tKY\tTrimble County\tH1\n40055\t21223\tPendleton\tKY\tTrimble County\tH1\n42459\t21225\tSturgis\tKY\tUnion County\tH1\n42437\t21225\tMorganfield\tKY\tUnion County\tH1\n42404\t21225\tClay\tKY\tUnion County\tH1\n42462\t21225\tWaverly\tKY\tUnion County\tH1\n42460\t21225\tSullivan\tKY\tUnion County\tH1\n42461\t21225\tUniontown\tKY\tUnion County\tH1\n42101\t21227\tBowling green\tKY\tWarren County\tH1\n42102\t21227\tBowling green\tKY\tWarren County\tH1\n42171\t21227\tSmiths grove\tKY\tWarren County\tH1\n42103\t21227\tBowling green\tKY\tWarren County\tH1\n42104\t21227\tBowling green\tKY\tWarren County\tH1\n42206\t21227\tAuburn\tKY\tWarren County\tH1\n42159\t21227\tOakland\tKY\tWarren County\tH1\n42122\t21227\tAlvaton\tKY\tWarren County\tH1\n42274\t21227\tRockfield\tKY\tWarren County\tH1\n42275\t21227\tRoundhill\tKY\tWarren County\tH1\n42170\t21227\tWoodburn\tKY\tWarren County\tH1\n40468\t21229\tPerryville\tKY\tWashington County\tH1\n40037\t21229\tLoretto\tKY\tWashington County\tH1\n40069\t21229\tSpringfield\tKY\tWashington County\tH1\n40061\t21229\tSaint catharine\tKY\tWashington County\tH1\n40033\t21229\tLebanon\tKY\tWashington County\tH1\n40008\t21229\tBloomfield\tKY\tWashington County\tH1\n40078\t21229\tWillisburg\tKY\tWashington County\tH1\n40342\t21229\tLawrenceburg\tKY\tWashington County\tH1\n40040\t21229\tMackville\tKY\tWashington County\tH1\n40330\t21229\tHarrodsburg\tKY\tWashington County\tH1\n42642\t21231\tRussell springs\tKY\tWayne County\tH1\n42602\t21231\tAlbany\tKY\tWayne County\tH1\n42603\t21231\tAlpha\tKY\tWayne County\tH1\n42633\t21231\tMonticello\tKY\tWayne County\tH1\n42544\t21231\tNancy\tKY\tWayne County\tH1\n42518\t21231\tBronston\tKY\tWayne County\tH1\n42437\t21233\tMorganfield\tKY\tWebster County\tH1\n42452\t21233\tRobards\tKY\tWebster County\tH1\n42450\t21233\tProvidence\tKY\tWebster County\tH1\n42455\t21233\tSebree\tKY\tWebster County\tH1\n42441\t21233\tNebo\tKY\tWebster County\tH1\n42404\t21233\tClay\tKY\tWebster County\tH1\n42463\t21233\tWheatcroft\tKY\tWebster County\tH1\n42444\t21233\tPoole\tKY\tWebster County\tH1\n42456\t21233\tSlaughters\tKY\tWebster County\tH1\n42409\t21233\tDixon\tKY\tWebster County\tH1\n42406\t21233\tCorydon\tKY\tWebster County\tH1\n40769\t21235\tWilliamsburg\tKY\tWhitley County\tH1\n40730\t21235\tEmlyn\tKY\tWhitley County\tH1\n40701\t21235\tCorbin\tKY\tWhitley County\tH1\n42635\t21235\tPine knot\tKY\tWhitley County\tH1\n40906\t21235\tBarbourville\tKY\tWhitley County\tH1\n40759\t21235\tRockholds\tKY\tWhitley County\tH1\n40771\t21235\tWoodbine\tKY\tWhitley County\tH1\n40741\t21235\tLondon\tKY\tWhitley County\tH1\n40763\t21235\tSiler\tKY\tWhitley County\tH1\n40940\t21235\tFrakes\tKY\tWhitley County\tH1\n41311\t21237\tBeattyville\tKY\tWolfe County\tH1\n41360\t21237\tPine ridge\tKY\tWolfe County\tH1\n41301\t21237\tCampton\tKY\tWolfe County\tH1\n41332\t21237\tHazel green\tKY\tWolfe County\tH1\n41365\t21237\tRogers\tKY\tWolfe County\tH1\n40383\t21239\tVersailles\tKY\tWoodford County\tH1\n40390\t21239\tWilmore\tKY\tWoodford County\tH1\n40347\t21239\tMidway\tKY\tWoodford County\tH1\n40513\t21239\tLexington\tKY\tWoodford County\tH1\n40601\t21239\tFrankfort\tKY\tWoodford County\tH1\n40510\t21239\tLexington\tKY\tWoodford County\tH1\n70543\t22001\tIota\tLA\tAcadia Parish\tH1\n70534\t22001\tEstherwood\tLA\tAcadia Parish\tH1\n70546\t22001\tJennings\tLA\tAcadia Parish\tH1\n70525\t22001\tChurch point\tLA\tAcadia Parish\tH1\n70559\t22001\tMorse\tLA\tAcadia Parish\tH1\n70537\t22001\tEvangeline\tLA\tAcadia Parish\tH1\n70526\t22001\tCrowley\tLA\tAcadia Parish\tH1\n70516\t22001\tBranch\tLA\tAcadia Parish\tH1\n70531\t22001\tEgan\tLA\tAcadia Parish\tH1\n70556\t22001\tMermentau\tLA\tAcadia Parish\tH1\n70535\t22001\tEunice\tLA\tAcadia Parish\tH1\n70578\t22001\tRayne\tLA\tAcadia Parish\tH1\n70529\t22001\tDuson\tLA\tAcadia Parish\tH1\n70515\t22001\tBasile\tLA\tAcadia Parish\tH1\n70583\t22001\tScott\tLA\tAcadia Parish\tH1\n70640\t22003\tFenton\tLA\tAllen Parish\tH1\n70662\t22003\tSugartown\tLA\tAllen Parish\tH1\n70638\t22003\tElizabeth\tLA\tAllen Parish\tH1\n70637\t22003\tDry creek\tLA\tAllen Parish\tH1\n70651\t22003\tLeblanc\tLA\tAllen Parish\tH1\n70658\t22003\tReeves\tLA\tAllen Parish\tH1\n70532\t22003\tElton\tLA\tAllen Parish\tH1\n70657\t22003\tRagley\tLA\tAllen Parish\tH1\n70644\t22003\tGrant\tLA\tAllen Parish\tH1\n70655\t22003\tOberlin\tLA\tAllen Parish\tH1\n70654\t22003\tMittie\tLA\tAllen Parish\tH1\n70656\t22003\tPitkin\tLA\tAllen Parish\tH1\n71463\t22003\tOakdale\tLA\tAllen Parish\tH1\n71433\t22003\tGlenmora\tLA\tAllen Parish\tH1\n70648\t22003\tKinder\tLA\tAllen Parish\tH1\n70346\t22005\tDonaldsonville\tLA\tAscension Parish\tH1\n70737\t22005\tGonzales\tLA\tAscension Parish\tH1\n70774\t22005\tSaint amant\tLA\tAscension Parish\tH1\n70769\t22005\tPrairieville\tLA\tAscension Parish\tH1\n70718\t22005\tBrittany\tLA\tAscension Parish\tH1\n70728\t22005\tDuplessis\tLA\tAscension Parish\tH1\n70734\t22005\tGeismar\tLA\tAscension Parish\tH1\n70778\t22005\tSorrento\tLA\tAscension Parish\tH1\n70449\t22005\tMaurepas\tLA\tAscension Parish\tH1\n70725\t22005\tDarrow\tLA\tAscension Parish\tH1\n70346\t22007\tDonaldsonville\tLA\tAssumption Parish\tH1\n70390\t22007\tNapoleonville\tLA\tAssumption Parish\tH1\n70372\t22007\tLabadieville\tLA\tAssumption Parish\tH1\n70393\t22007\tPlattenville\tLA\tAssumption Parish\tH1\n70380\t22007\tMorgan city\tLA\tAssumption Parish\tH1\n70341\t22007\tBelle rose\tLA\tAssumption Parish\t
